vi "MovingAvg.vi"(11 "Raw Voltage Input [Int.]":i64) -> (3 "Analog Volt Out [FXP.]":fxp<+/-,22,5>)   [LabVIEW 2018, in "FPGA functions.lvlib"]
doc: "Moving average - 320 points \n\nOutput is in fixed point output."
uses:
  FPGA functions.lvlib
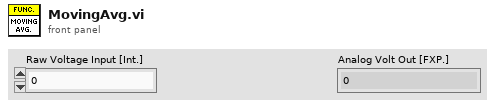
[diagram p1: front panel]
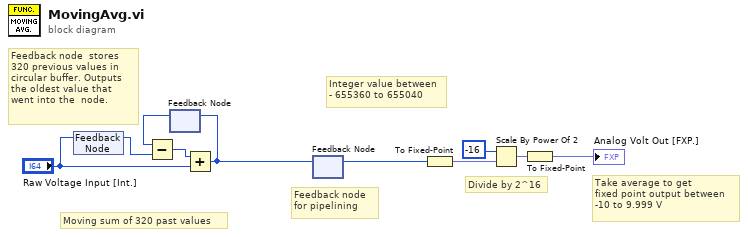
[diagram p0: block diagram]
diagram:
  # "Feedback node  stores \n320 previous values in \ncircular buffer. Outputs \nthe oldest value that \nwent into the  node."
  # "Feedback node \nfor pipelining"
  # "Divide by 2^16"
  # "Integer value between\n- 655360 to 655040"
  # "Take average to get \nfixed point output between\n-10 to 9.999 V"
  # "Moving sum of 320 past values"
  n1 = feedback-in #1("Raw Voltage Input [Int.]") -> ()
  n2 = feedback #1() -> (w8:i64)  [unwired: 1 in]
  n3 = feedback #2() -> (w9:i64)  [unwired: 1 in]
  n4 = Subtract(x=w9, y=w8) -> (x-y=w10:i64)
  n5 = Add(x=w10, y="Raw Voltage Input [Int.]") -> (x+y=w1:i64)
  n6 = feedback-in #2(w1) -> ()
  n7 = feedback-in #3(w1) -> ()
  n8 = feedback #3() -> (w3:i64)  [unwired: 1 in]
  n9 = To Fixed-Point(number=w3) -> (fixed-point=w5:fxp<+/-,38,21>)  [unwired: 1 out]
  n10 = Scale By Power Of 2(n=-16, x=w5) -> (x*2^n=w4:fxp<+/-,38,21>)
  n11 = To Fixed-Point(number=w4) -> (fixed-point=→"Analog Volt Out [FXP.]":fxp<+/-,22,5>)  [unwired: 1 out]
